vi "build_commands_rabi.vi"(8 "Refocus_s":u32, 9 "Refocus?":bool, 11 "Rabi_parameters":T1) -> (1 "commands":T2(array[cluster]))   [LabVIEW 2018]
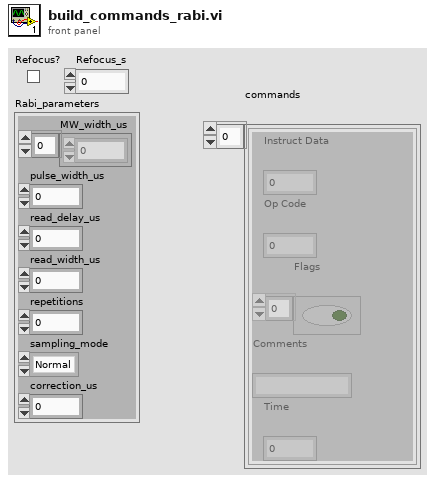
[diagram p1: front panel]
types:
  T1 = cluster{"MW_width_us":dbl[], "pulse_width_us":dbl, "read_delay_us":dbl, "read_width_us":dbl, "repetitions":i32, "sampling_mode":enum16{"Normal", "Sweep"}, "correction_us":dbl}
  T2 = cluster{"Instruct Data":i32, "Op Code":i32, "Flags":bool[], "Comments":string, "Time":dbl}[]
  T3 = cluster{"Instruct Data":i32, "Op Code":i32, "Flags":bool[], "Comments":string, "Time":dbl}
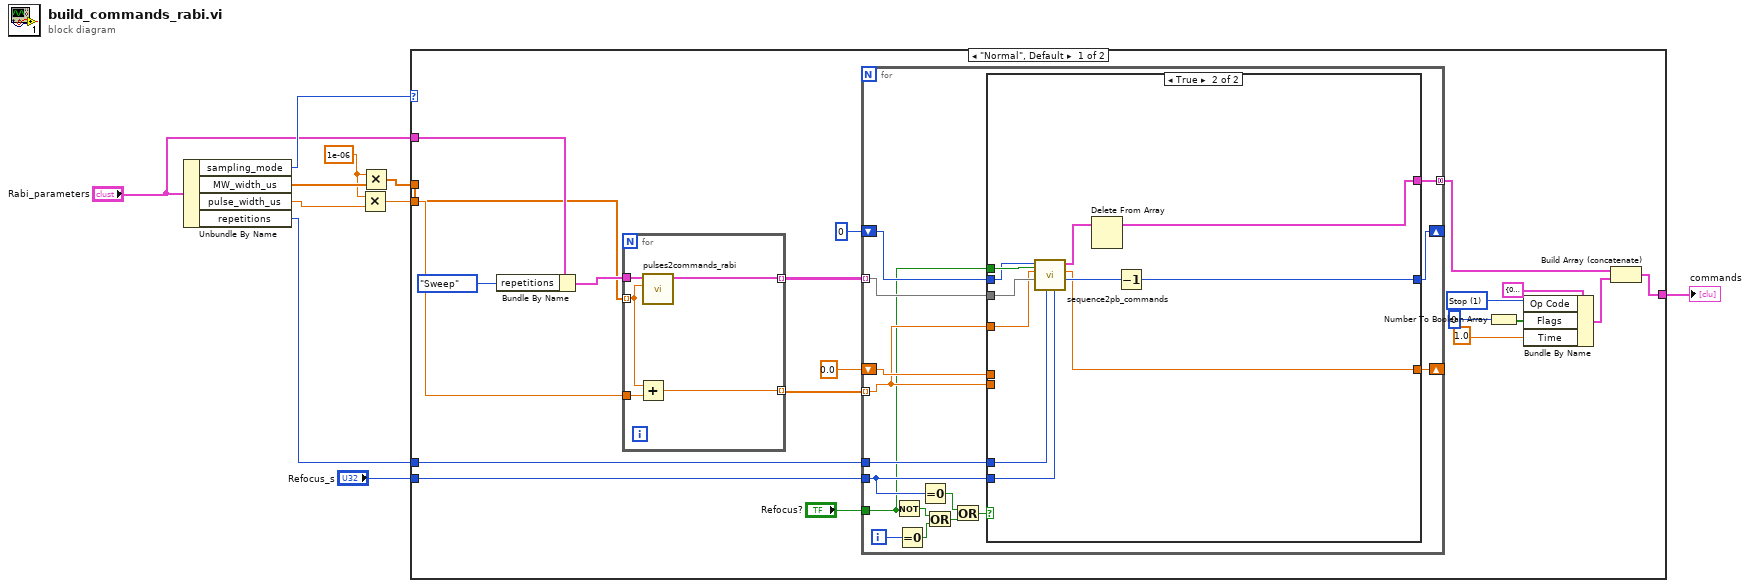
[diagram p0: block diagram]
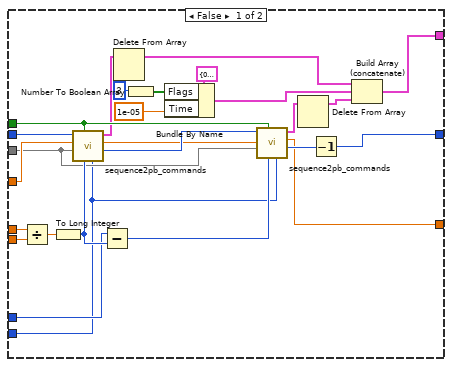
[diagram p2: hidden frame]
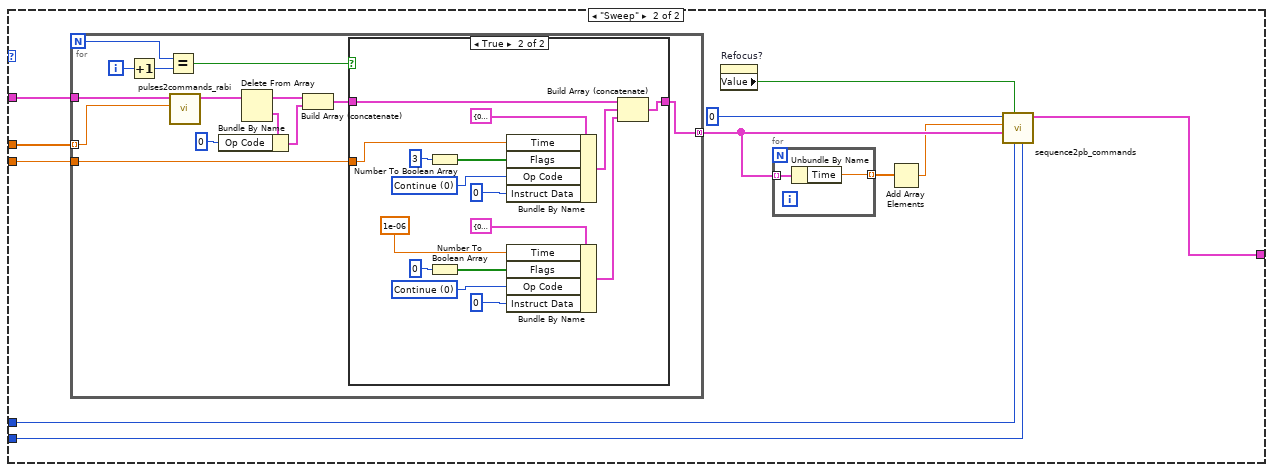
[diagram p3: hidden frame]
diagram:
  w2 = 1e-06
  n1 = Unbundle By Name("Rabi_parameters") -> ("sampling_mode"=w10:enum16{"Normal", "Sweep"}, "MW_width_us"=w5:dbl[], "pulse_width_us"=w3:dbl, "repetitions"=w6:i32)
  n2 = Multiply(x=w2, y=w3) -> (x*y=w1:dbl)
  n3 = Multiply(x=w2, y=w5) -> (x*y=w4:dbl[])
  n4 = case shown="\"Normal\", Default" w10 {
    tunnel: w1 -> [w28 w99]
    tunnel: w4 -> [w20 w98]
    tunnel: w6 -> [w19 w96]
    tunnel: [w11 w93] -> w9
    tunnel: "Refocus_s" -> [w23 w95]
    tunnel: "Rabi_parameters" -> [w21 w92]
    frame "Normal", Default {
      w13 = 1 items=["Continue", "Stop", "Loop", "End Loop", "JSR", "RTS", "Branch", "Long Delay", "Wait"] ("Op Code 2")
      n5 = Bundle By Name(cluster=w21, "repetitions"=enum16{"Normal", "Sweep"}."Sweep" ("Sampling mode")) -> (w29:T1)
      n6 = for {
        tunnel: w29 -> [w88]
        tunnel: w20 -> [w86] mode=indexing
        tunnel: [w87] -> w25 mode=indexing
        tunnel: w28 -> [w85]
        tunnel: [w84] -> w26 mode=indexing
        n7 = Add(x=w86, y=w85) -> (x+y=w84:dbl)
        n8 = call "pulses2commands_rabi.vi"("MW_width"=w86, "Rabi_parameters"=w88) -> ("Array out"=w87:T2)  [unwired: 9 in]
      }
      n9 = for {
        shift-right: [w33] -> _
        shift-left: 0 -> [w39]
        tunnel: w26 -> [w38] mode=indexing
        tunnel: w25 -> [w37] mode=indexing
        tunnel: "Refocus?" -> [w34]
        tunnel: w23 -> [w36]
        shift-right: [w32] -> _
        shift-left: 0.0 -> [w40]
        tunnel: w19 -> [w35]
        tunnel: [w31] -> w12 mode=concatenating
        i -> [w46]
        n10 = Not(x=w34) -> (.not. x?=w44:bool)
        n11 = Equal To 0?(x=w46) -> (x = 0?=w45:bool)
        n12 = Equal To 0?(x=w36) -> (x = 0?=w42:bool)
        n13 = Or(x=w44, y=w45) -> (x .or. y?=w43:bool)
        n14 = Or(x=w42, y=w43) -> (x .or. y?=w41:bool)
        n15 = case shown="True" w41 {
          tunnel: w40 -> [w72 _]
          tunnel: w38 -> [w71 _]
          tunnel: w39 -> [w69 w77]
          tunnel: w38 -> [w68 w73]
          tunnel: w37 -> [w65 w74]
          tunnel: w36 -> [w63 w76]
          tunnel: w35 -> [w66 w75]
          tunnel: w34 -> [w62 w78]
          tunnel: [w54 w82] -> w33
          tunnel: [w53 w81] -> w32
          tunnel: [w49 w79] -> w31
          frame False {
            n16 = Divide(x=w72, y=w71) -> (x/y=w70:dbl)
            n17 = To Long Integer(number=w70) -> (32bit integer=w67:i32)
            n18 = call "sequence2pb_commands.vi"("Refocus_s"=w63, "Repetitions"=w67, "Refocus?"=w62, "command_sequence"=w65, "Sequence_length"=w68, "start_command"=w69) -> ("end_command"=w61:i32, "t_remaining"=w60:dbl, "PB_commands"=w59:T2)  [unwired: 3 in]
            n19 = Subtract(x=w66, y=w67) -> (x-y=w64:i32)
            n20 = Delete From Array(array=w59) -> (array with subset deleted=w47:T2)  [unwired: 2 in, 1 out]
            n21 = Number To Boolean Array(number=3) -> (Boolean array=w56:bool[])
            n22 = Bundle By Name(cluster=T3 {"Instruct Data"=0, "Op Code"=0, "Flags"=[FALSE, FALSE, FALSE, FALSE, FALSE, FALSE, FALSE, FALSE, FALSE, FALSE, FALSE, FALSE, FALSE, FALSE, FALSE, FALSE, FALSE, FALSE, FALSE, FALSE, FALSE, FALSE, FALSE, FALSE], "Comments"="", "Time"=1e-06} ("PB Instruction"), "Flags"=w56, "Time"=1e-05) -> (w50:T3)
            n23 = call "sequence2pb_commands.vi"("Refocus_s"=w63, "Repetitions"=w64, "Refocus?"=w62, "command_sequence"=w65, "Sequence_length"=w60, "start_command"=w61) -> ("end_command"=w55:i32, "t_remaining"=w53:dbl, "PB_commands"=w52:T2)  [unwired: 3 in]
            n24 = Delete From Array(array=w52) -> (array with subset deleted=w51:T2)  [unwired: 2 in, 1 out]
            n25 = Decrement(x=w55) -> (x-1=w54:i32)
            n26 = Build Array (concatenate)(w47, w50, w51) -> (w49:T2)
          }
          frame True {
            n27 = call "sequence2pb_commands.vi"("Refocus_s"=w76, "Repetitions"=w75, "Refocus?"=w78, "command_sequence"=w74, "Sequence_length"=w73, "start_command"=w77) -> ("end_command"=w83:i32, "t_remaining"=w81:dbl, "PB_commands"=w80:T2)  [unwired: 3 in]
            n28 = Delete From Array(array=w80) -> (array with subset deleted=w79:T2)  [unwired: 2 in, 1 out]
            n29 = Decrement(x=w83) -> (x-1=w82:i32)
          }
        }
      }
      n30 = Number To Boolean Array(number=0) -> (Boolean array=w17:bool[])
      n31 = Bundle By Name(cluster=T3 {"Instruct Data"=0, "Op Code"=0, "Flags"=[FALSE, FALSE, FALSE, FALSE, FALSE, FALSE, FALSE, FALSE, FALSE, FALSE, FALSE, FALSE, FALSE, FALSE, FALSE, FALSE, FALSE, FALSE, FALSE, FALSE, FALSE, FALSE, FALSE, FALSE], "Comments"="", "Time"=1e-06} ("PB Instruction"), "Op Code"=w13, "Flags"=w17, "Time"=1.0) -> (w15:T3)
      n32 = Build Array (concatenate)(w12, w15) -> (w11:T2)
    }
    frame "Sweep" {
      n33 = for {
        N -> [w107]
        tunnel: w99 -> [w104]
        tunnel: w98 -> [w102] mode=indexing
        tunnel: [w110] -> w91 mode=concatenating
        tunnel: w92 -> [w103]
        i -> [w109]
        n34 = Increment(x=w109) -> (x+1=w108:i32)
        n35 = Equal?(x=w107, y=w108) -> (x = y?=w106:bool)
        n36 = call "pulses2commands_rabi.vi"("MW_width"=w102, "Rabi_parameters"=w103) -> ("Array out"=w105:T2)  [unwired: 9 in]
        n37 = Delete From Array(array=w105) -> (deleted portion=w115:T3, array with subset deleted=w112:T2)  [unwired: 2 in]
        n38 = Bundle By Name(cluster=w115, "Op Code"=0) -> (w113:T3)
        n39 = Build Array (concatenate)(w112, w113) -> (w111:T2)
        n40 = case shown="True" w106 {
          tunnel: w111 -> [w116 w132]
          tunnel: [w116 w131] -> w110
          tunnel: w104 -> [_ w118]
          frame False {
          }
          frame True {
            w124 = 0 items=["Continue", "Stop", "Loop", "End Loop", "JSR", "RTS", "Branch", "Long Delay", "Wait"] ("Op Code 2")
            w130 = 0 items=["Continue", "Stop", "Loop", "End Loop", "JSR", "RTS", "Branch", "Long Delay", "Wait"] ("Op Code 2")
            n41 = Number To Boolean Array(number=3) -> (Boolean array=w121:bool[])
            n42 = Number To Boolean Array(number=0) -> (Boolean array=w127:bool[])
            n43 = Bundle By Name(cluster=T3 {"Instruct Data"=0, "Op Code"=0, "Flags"=[FALSE, FALSE, FALSE, FALSE, FALSE, FALSE, FALSE, FALSE, FALSE, FALSE, FALSE, FALSE, FALSE, FALSE, FALSE, FALSE, FALSE, FALSE, FALSE, FALSE, FALSE, FALSE, FALSE, FALSE], "Comments"="", "Time"=1e-06} ("PB Instruction"), "Time"=w118, "Flags"=w121, "Op Code"=w124, "Instruct Data"=0) -> (w119:T3)
            n44 = Bundle By Name(cluster=T3 {"Instruct Data"=0, "Op Code"=0, "Flags"=[FALSE, FALSE, FALSE, FALSE, FALSE, FALSE, FALSE, FALSE, FALSE, FALSE, FALSE, FALSE, FALSE, FALSE, FALSE, FALSE, FALSE, FALSE, FALSE, FALSE, FALSE, FALSE, FALSE, FALSE], "Comments"="", "Time"=1e-06} ("PB Instruction"), "Time"=1e-06, "Flags"=w127, "Op Code"=w130, "Instruct Data"=0) -> (w125:T3)
            n45 = Build Array (concatenate)(w132, w119, w125) -> (w131:T2)
          }
        }
      }
      n46 = property on="Refocus?" class="Bool (strict)"() -> ("Value"=w94:bool)  [unwired: 2 in, 2 out]
      n47 = for {
        tunnel: w91 -> [w101] mode=indexing
        tunnel: [w100] -> w90 mode=indexing
        n48 = Unbundle By Name(w101) -> ("Time"=w100:dbl)
      }
      n49 = Add Array Elements(numeric array=w90) -> (sum=w89:dbl)
      n50 = call "sequence2pb_commands.vi"("Refocus_s"=w95, "Repetitions"=w96, "Refocus?"=w94, "command_sequence"=w91, "Sequence_length"=w89, "start_command"=0) -> ("PB_commands"=w93:T2)  [unwired: 3 in, 2 out]
    }
  }
  "commands" <- w9
